vi "Header.vi"(2 "23BitData":u32 format="%024b", 4 "1BitHeaderIndex":u8 format="%08b", 5 "8BitHead":u8 format="%08b") -> (0 "32BitOutput":u32 format="%032b")   [LabVIEW 2014]
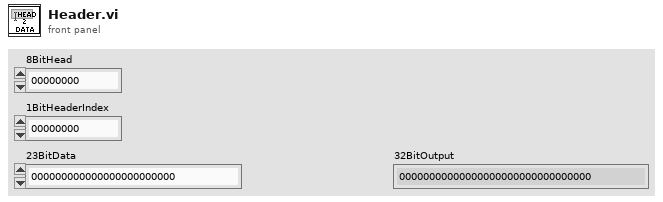
[diagram p1: front panel]
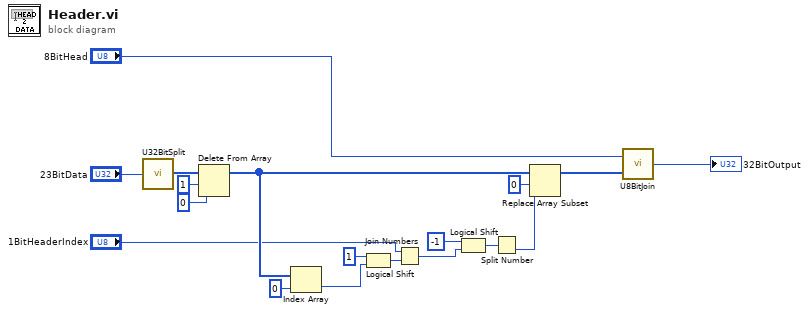
[diagram p0: block diagram]
diagram:
  n1 = call "U32BitSplit.vi"("U32"="23BitData") -> ("U8 Array"=w15:u8[])
  n2 = Delete From Array(array=w15, length=1, index=0) -> (array with subset deleted=w13:u8[])  [unwired: 1 out]
  n3 = Index Array(array=w13, index=0) -> (element=w7:u8)
  n4 = Logical Shift(y=i16 1, x=w7) -> (x << y=w2:u8)
  n5 = Join Numbers(hi="1BitHeaderIndex", lo=w2) -> ((hi.lo)=w4:u16)
  n6 = Logical Shift(y=i16 -1, x=w4) -> (x << y=w5:u16)
  n7 = Split Number(x=w5) -> (lo(x)=w1:u8)  [unwired: 1 out]
  n8 = Replace Array Subset(array=w13, new element=w1, index=0) -> (w10:u8[])
  n9 = call "U8BitJoin.vi"("array"=w10, "hi"="8BitHead") -> ("U32"=→"32BitOutput":u32)
